vi "PCIeDiffractiveTest.vi"() -> ()   [LabVIEW 2017]
uses:
  <vilib>/Utility/file.llb/Write To Spreadsheet File (I64).vi
  Blink_C_wrapper.dll
  ImageGen.dll
panel:
  out "Array":u8[][](array[numeric])
  out "BoardNum":i32
  # "PCIe  LabVIEWSDK"
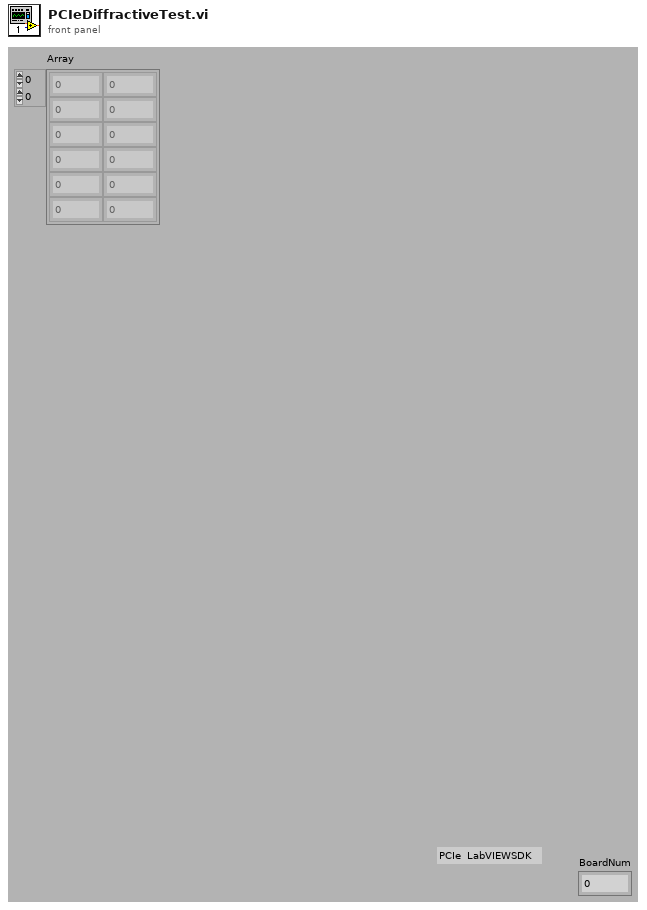
[diagram p1: front panel]
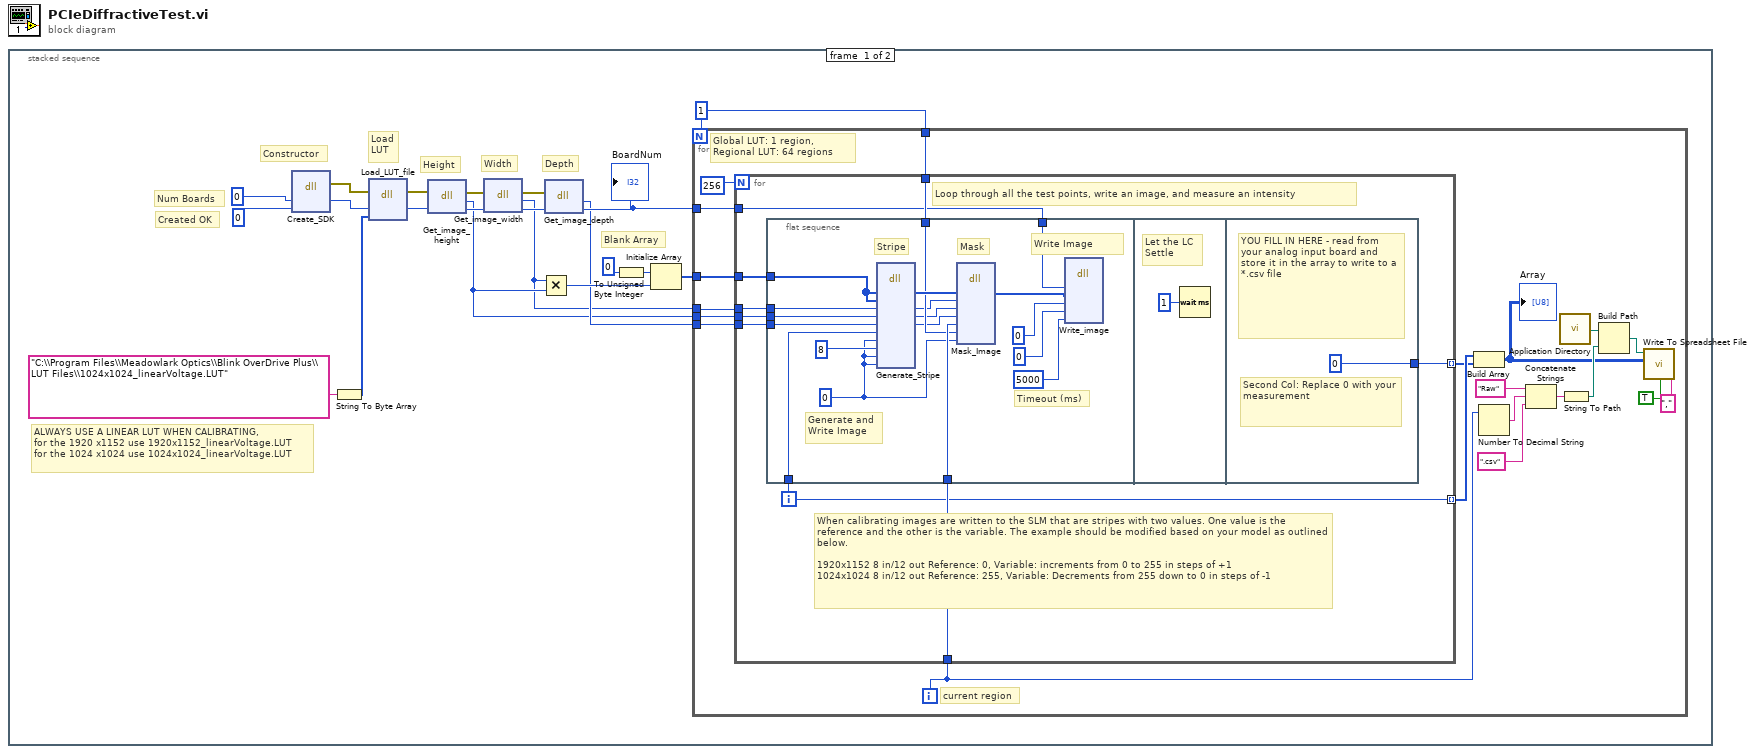
[diagram p0: block diagram]
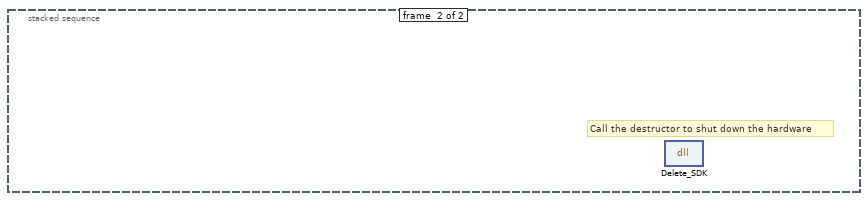
[diagram p2: hidden frame]
diagram:
  n1 = stacked-sequence {
    frame #0 {
      w9 = 1
      # "Num Boards"
      # "Depth"
      # "Blank Array"
      # "Width"
      # "Height"
      # "ALWAYS USE A LINEAR LUT WHEN CALIBRATING,\nfor the 1920 x1152 use 1920x1152_linearVoltage.LUT\nfor the 1024 x1024 use 1024x1024_linearVoltage.LUT"
      # "Load\nLUT"
      # "Created OK"
      # "Constructor"
      n2 = dll-call lib="C:/Meadowlark/Repos-git/MeadowlarkOverdrivePlus/src/Blink_SDK_example/Blink_C_wrapper.dll" fn="Create_SDK"("n_boards_found"=0, "constructed_ok"=0) -> (error out=w20:errorcluster, "n_boards_found"=w17:u64)  [unwired: 5 in, 1 out]
      n3 = String To Byte Array(string="C:\\Program Files\\Meadowlark Optics\\Blink OverDrive Plus\\LUT Files\\1024x1024_linearVoltage.LUT") -> (unsigned byte array=w19:u8[])
      n4 = dll-call lib="C:/Meadowlark/Repos-git/MeadowlarkOverdrivePlus/src/Blink_SDK_example/Blink_C_wrapper.dll" fn="Load_LUT_file"(error in=w20, "Board"=w17, "LUTPath"=w19) -> (error out=w14:errorcluster, "Board"=w16:u32)  [unwired: 4 in, 1 out]
      n5 = dll-call lib="C:/Meadowlark/Repos-git/MeadowlarkOverdrivePlus/src/Blink_SDK_example/Blink_C_wrapper.dll" fn="Get_image_height"(error in=w14, "Board"=w16) -> (error out=w13:errorcluster, "return type"=w2:i32, "Board"=w15:u32)  [unwired: 2 in, 1 out]
      n6 = dll-call lib="C:/Meadowlark/Repos-git/MeadowlarkOverdrivePlus/src/Blink_SDK_example/Blink_C_wrapper.dll" fn="Get_image_width"(error in=w13, "Board"=w15) -> (error out=w7:errorcluster, "return type"=w1:i32, "Board"=w6:u32)  [unwired: 2 in, 1 out]
      n7 = Multiply(x=w1, y=w2) -> (x*y=w8:i32)
      n8 = dll-call lib="C:/Meadowlark/Repos-git/MeadowlarkOverdrivePlus/src/Blink_SDK_example/Blink_C_wrapper.dll" fn="Get_image_depth"(error in=w7, "Board"=w6) -> ("return type"=w4:i32, "Board"=w5:u32)  [unwired: 2 in, 2 out]
      "BoardNum" <- w5
      n9 = To Unsigned Byte Integer(number=0) -> (unsigned 8bit integer=w12:u8)
      n10 = Initialize Array(w12, w8) -> (w10:u8[])
      n11 = for {
        N: w9 -> [_]
        tunnel: w10 -> [w41]
        tunnel: w2 -> [w40]
        tunnel: w1 -> [w39]
        tunnel: w9 -> [w37]
        tunnel: w5 -> [w23]
        tunnel: w4 -> [w22]
        i -> [w35]
        # "Global LUT: 1 region, Regional LUT: 64 regions"
        # "current region"
        n12 = for {
          N: 256 -> [_]
          tunnel: w41 -> [w50]
          tunnel: w40 -> [w49]
          tunnel: w39 -> [w48]
          tunnel: w35 -> [w47]
          tunnel: w37 -> [w46]
          tunnel: [w45] -> w25 mode=indexing
          tunnel: [w44] -> w24 mode=indexing
          tunnel: w23 -> [w43]
          tunnel: w22 -> [w42]
          i -> [w45]
          # "When calibrating images are written to the SLM that are stripes with two values. One value is the reference and the other is the variable. The example should be modified based on your model as outlined below.\n \n1920x1152 8 in/12 out Reference: 0, Variable: increments from 0 to 255 in steps of +1 \n1024x1024 8 in/12 out Reference: 255, Variable: Decrements from 255 down to 0 in steps of -1"
          # "Loop through all the test points, write an image, and measure an intensity"
          n13 = flat-sequence {
            tunnel: w50 -> [w54]
            tunnel: w49 -> [w55]
            tunnel: w48 -> [w56]
            tunnel: w47 -> [w67]
            tunnel: w46 -> [w66]
            tunnel: w45 -> [w62]
            tunnel: w43 -> [w58]
            tunnel: w42 -> [w53]
            tunnel: [0] -> w44
            frame #0 {
              w51 = 0
              # "Timeout (ms)"
              # "Write Image"
              # "Generate and \nWrite Image"
              # "Mask"
              # "Stripe"
              n14 = dll-call lib="C:/Meadowlark/Repos-git/MeadowlarkOverdrivePlus/src/Blink_SDK_example/ImageGen.dll" fn="Generate_Stripe"("Array"=w54, "WFC"=w54, "Width"=w56, "Height"=w55, "Depth"=w53, "PixelValOne"=w62, "PixelValTwo"=w51, "PixelsPerStripe"=8, "Vertical"=w51, "RGB"=w51) -> ("Array"=w68:u8[], "Width"=w64:i32, "Height"=w65:i32, "Depth"=w52:i32)  [unwired: 10 in, 2 out]
              n15 = dll-call lib="C:/Meadowlark/Repos-git/MeadowlarkOverdrivePlus/src/Blink_SDK_example/ImageGen.dll" fn="Mask_Image"("Array"=w68, "Width"=w64, "Height"=w65, "Depth"=w52, "Region"=w67, "NumRegions"=w66, "RGB"=w51) -> ("Array"=w59:u8[])  [unwired: 10 in, 2 out]
              n16 = dll-call lib="C:/Meadowlark/Repos-git/MeadowlarkOverdrivePlus/src/Blink_SDK_example/Blink_C_wrapper.dll" fn="Write_image"("board"=w58, "Image"=w59, "WaitForTrigger"=0, "OutputPulseImageFlip"=0, "timeout"=5000) -> ()  [unwired: 9 in, 2 out]
            }
            frame #1 {
              # "Let the LC \nSettle"
              n17 = Wait (ms)(milliseconds to wait=u32 1) -> ()  [unwired: 1 out]
            }
            frame #2 {
              # "Second Col: Replace 0 with your measurement"
              # "YOU FILL IN HERE - read from  your analog input board and store it in the array to write to a *.csv file"
            }
          }
        }
        n18 = Build Array(w25, w24) -> (w26:i32[][])
        "Array" <- w26
        n19 = Number To Decimal String(number=w35) -> (decimal integer string=w34:string)  [unwired: 1 in]
        n20 = Concatenate Strings("Raw", w34, ".csv") -> (w32:string)
        n21 = call <vilib>:"Application Directory.vi"() -> ("Application Directory"=w31:path)
        n22 = String To Path(string=w32) -> (path=w30:path)
        n23 = Build Path(base path=w31, name or relative path=w30) -> (appended path=w29:path)
        n24 = call-poly <vilib>:"Write To Spreadsheet File.vi"("delimiter (\\t)"=",", "transpose? (no:F)"=TRUE, "2D data"=w26, "file path (dialog if empty)"=w29) -> ()  [unwired: 4 in, 1 out]
      }
    }
    frame #1 {
      # "Call the destructor to shut down the hardware"
      n25 = dll-call lib="C:/Meadowlark/Repos-git/MeadowlarkOverdrivePlus/src/Blink_SDK_example/Blink_C_wrapper.dll" fn="Delete_SDK"() -> ()  [unwired: 4 in, 2 out]
    }
  }
